vi "Trigger Parameters FG.vi"(7 "Action":T1, 8 "error in (no error)":errorcluster, 10 "Trigger Parameters":T3, 11 "Item Ref in":T2 format="%.0x") -> (0 "error out":errorcluster={"status"=TRUE, "code"=1172, "source"="Invoke Node Error calling static method NationalInstruments.VeriStand.SystemDefinitionAPI.NodeIDUtil.IDToCustomDeviceBase, (System.Reflection.TargetInvocationException: Exception has been thrown by the target of an invocation.\n\tInner Exception: System.Exception: NI VeriStand Error: 36, The specified Item Ref is invalid. The Item Ref refers to an item that doesn't exist) <append><b>System.Exception</b> in Custom Device Offline API.lvlib:ID To Custom Device Base.vi->Custom Device Offline API.lvlib:Get Item Property (Variant).vi->Custom Device API.lvlib:Get Item Property (Variant).vi->Instrument Addon Shared.lvlib:Response Parameters FG.vi"}, 2 "Trigger Parameters":T3, 3 "Item Ref out":T2 format="%.0x")   [LabVIEW 2020, in "Instrument Addon Shared.lvlib"]
uses:
  Instrument Addon Shared.lvlib
  Trigger Parameters.ctl
  <vilib>/NI VeriStand/Custom Device API/Custom Device Item Ref.ctl
  FG Control.ctl
  Constants.vi
  <vilib>/NI VeriStand/Custom Device API/Get Item Property (Boolean).vi
  <vilib>/NI VeriStand/Custom Device API/Get Item Property (String).vi
  <vilib>/NI VeriStand/Custom Device API/Set Item Property (Boolean).vi
  <vilib>/NI VeriStand/Custom Device API/Set Item Property (String).vi
  <vilib>/NI VeriStand/Custom Device API/Custom Device API.lvlib
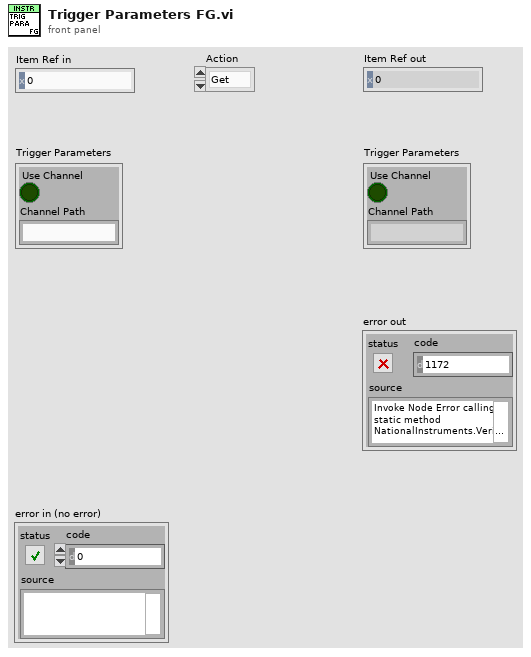
[diagram p1: front panel]
types:
  T1 = typedef "Instrument Addon Shared.lvlib/FG Control.ctl" = enum16{"Get", "Set"}
  T2 = typedef "Custom Device API.lvlib/Custom Device Item Ref.ctl" = u64
  T3 = typedef "Instrument Addon Shared.lvlib/Trigger Parameters.ctl" = cluster{"Use Channel":bool, "Channel Path":string}
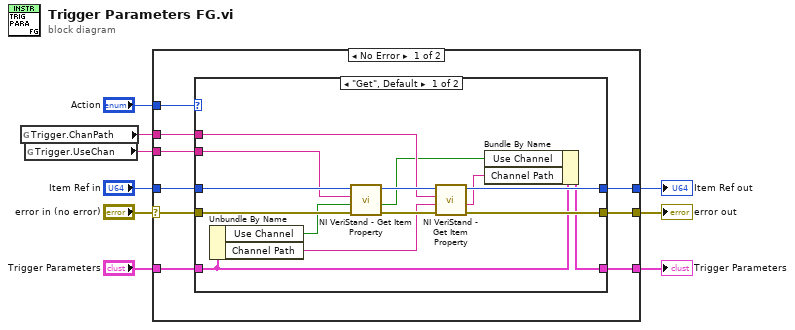
[diagram p0: block diagram]
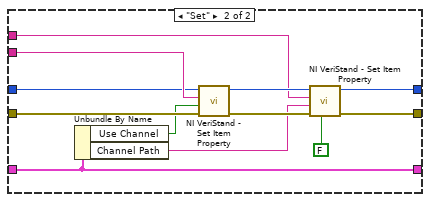
[diagram p2: hidden frame]
diagram:
  n1 = global read "Constants.vi" "Trigger.ChanPath"() -> (w1:string)
  n2 = global read "Constants.vi" "Trigger.UseChan"() -> (w3:string)
  n3 = case shown="No Error" "error in (no error)" {
    selector: "error in (no error)" -> [w13 w47]
    tunnel: w3 -> [w18 _]
    tunnel: [w17 w45] -> w7
    tunnel: "Item Ref in" -> [w16 w45]
    tunnel: "Trigger Parameters" -> [w15 w46]
    tunnel: [w14 w47] -> w6
    tunnel: [w12 w46] -> w2
    tunnel: "Action" -> [w11 _]
    tunnel: w1 -> [w10 _]
    frame No Error {
      n4 = case shown="\"Get\", Default" w11 {
        tunnel: w18 -> [w30 w44]
        tunnel: [w25 w38] -> w17
        tunnel: w16 -> [w31 w43]
        tunnel: w15 -> [w22 w36]
        tunnel: [w27 w39] -> w14
        tunnel: w13 -> [w32 w42]
        tunnel: [w21 w36] -> w12
        tunnel: w10 -> [w23 w37]
        frame "Get", Default {
          n5 = Unbundle By Name(w22) -> ("Use Channel"=w29:bool, "Channel Path"=w24:string)
          n6 = call-poly <vilib>:"NI VeriStand - Get Item Property.vi"("error in (no error)"=w32, "Default Value"=w29, "Property Name"=w30, "Item Ref in"=w31) -> ("error out"=w28:errorcluster, "Value"=w20:bool, "Item Ref out"=w26:T2)  [unwired: 4 in, 1 out]
          n7 = call-poly <vilib>:"NI VeriStand - Get Item Property.vi"("error in (no error)"=w28, "Default Value"=w24, "Property Name"=w23, "Item Ref in"=w26) -> ("error out"=w27:errorcluster, "Value"=w19:string, "Item Ref out"=w25:T2)  [unwired: 4 in, 1 out]
          n8 = Bundle By Name(cluster=w22, "Use Channel"=w20, "Channel Path"=w19) -> (w21:T3)
        }
        frame "Set" {
          n9 = Unbundle By Name(w36) -> ("Use Channel"=w35:bool, "Channel Path"=w34:string)
          n10 = call-poly <vilib>:"NI VeriStand - Set Item Property.vi"("error in (no error)"=w42, "Value"=w35, "Property Name"=w44, "Item Ref in"=w43) -> ("error out"=w40:errorcluster, "Item Ref out"=w41:T2)  [unwired: 5 in, 1 out]
          n11 = call-poly <vilib>:"NI VeriStand - Set Item Property.vi"("Binary String (T)"=FALSE, "error in (no error)"=w40, "Value"=w34, "Property Name"=w37, "Item Ref in"=w41) -> ("error out"=w39:errorcluster, "Item Ref out"=w38:T2)  [unwired: 4 in, 1 out]
        }
      }
    }
    frame Error {
    }
  }
  "error out" <- w6
  "Trigger Parameters" <- w2
  "Item Ref out" <- w7
